vi "WhichGoalVisible.vi"(0 "Goal Measurements":dbl[][](array[numeric]), 1 "No. of Goals":i32) -> (2 "Goal A":cluster{"X":dbl, "Y":dbl, "Dist":dbl}, 3 "Goal B":cluster{"X":dbl, "Y":dbl, "Dist":dbl}, 4 "Goal C":cluster{"X":dbl, "Y":dbl, "Dist":dbl})   [LabVIEW 2015]
uses:
  Robot Global Data.vi
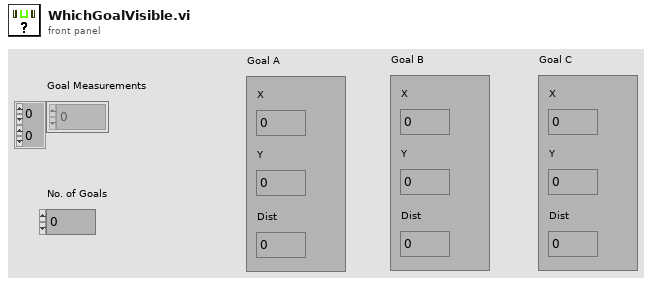
[diagram p1: front panel]
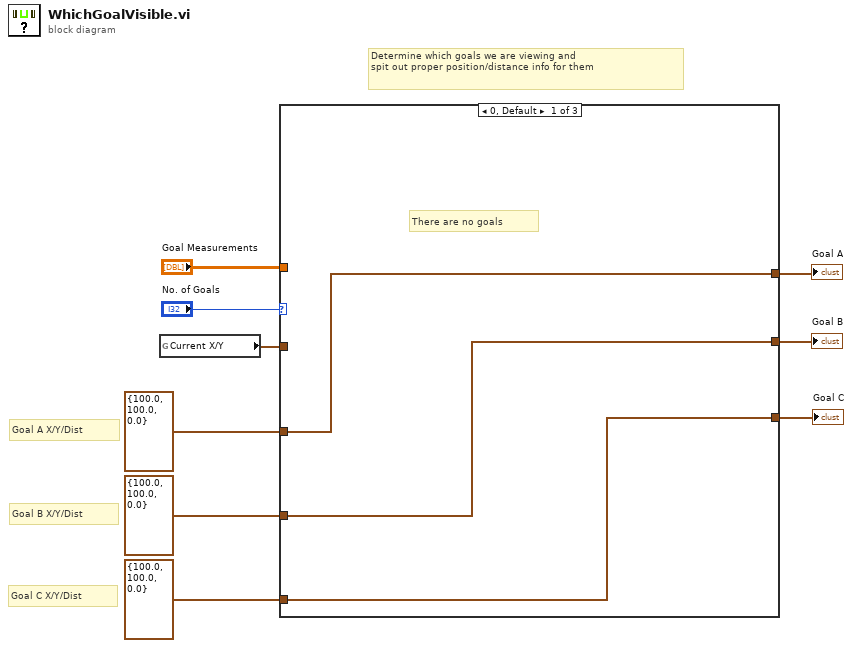
[diagram p0: block diagram]
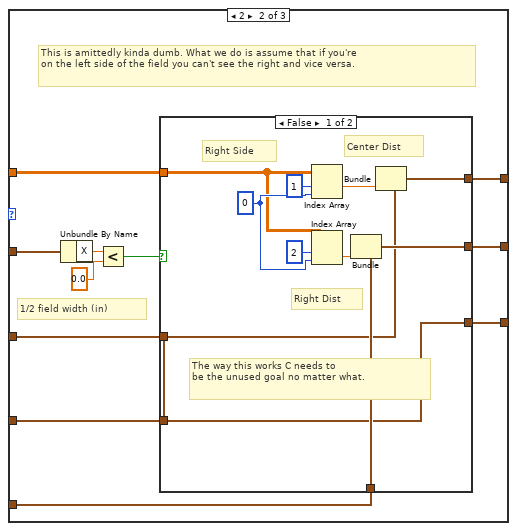
[diagram p2: hidden frame]
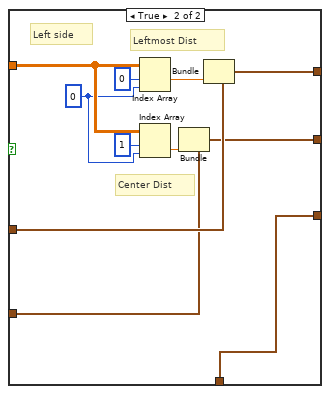
[diagram p3: hidden frame]
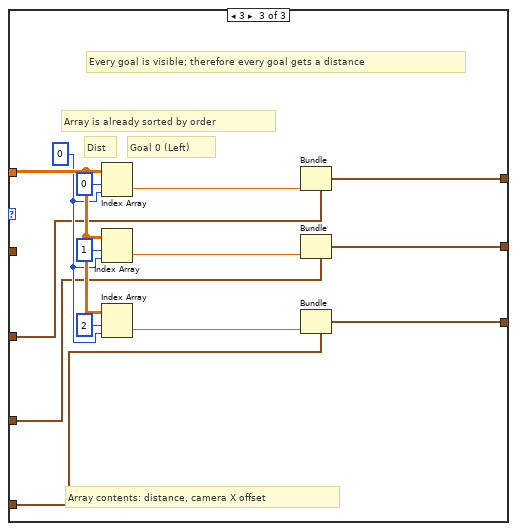
[diagram p4: hidden frame]
diagram:
  # "Determine which goals we are viewing and\nspit out proper position/distance info for them"
  # "Goal C X/Y/Dist"
  # "Goal B X/Y/Dist"
  # "Goal A X/Y/Dist"
  n1 = global read "Robot Global Data.vi" "Current X/Y"() -> (w1:cluster{"X":dbl, "Y":dbl})
  n2 = case shown="0, Default" "No. of Goals" {
    tunnel: [w12 w14 w55] -> w8
    tunnel: [w11 w15 w54] -> w7
    tunnel: [w10 w13 w52] -> w6
    tunnel: "Goal Measurements" -> [_ w16 w58]
    tunnel: cluster{dbl, dbl, dbl} {100.0, 100.0, 0.0} -> [w12 w19 w48]
    tunnel: cluster{dbl, dbl, dbl} {100.0, 100.0, 0.0} -> [w11 w18 w47]
    tunnel: cluster{dbl, dbl, dbl} {100.0, 100.0, 0.0} -> [w10 w17 w46]
    tunnel: w1 -> [_ w23 _]
    frame 0, Default {
      # "There are no goals"
    }
    frame 2 {
      # "This is amittedly kinda dumb. What we do is assume that if you're\non the left side of the field you can't see the right and vice versa."
      # "1/2 field width (in)"
      n3 = Unbundle By Name(w23) -> ("X"=w22:dbl)
      n4 = Less?(x=w22, y=0.0) -> (x < y?=w20:bool)
      n5 = case shown="False" w20 {
        tunnel: w19 -> [_ w40]
        tunnel: w18 -> [w24 w37]
        tunnel: w17 -> [w28 w34]
        tunnel: w16 -> [w27 w44]
        tunnel: [w25 w36] -> w15
        tunnel: [w26 w35] -> w14
        tunnel: [w24 w34] -> w13
        frame False {
          w31 = 0 ("index (row)")
          # "The way this works C needs to\nbe the unused goal no matter what."
          # "Center Dist"
          # "Right Dist"
          # "Right Side"
          n6 = Index Array(array=w27, index (row)=1, index (col)=w31) -> (element=w30:dbl)
          n7 = Index Array(array=w27, index (row)=2, index (col)=w31) -> (element=w29:dbl)
          n8 = Bundle(cluster=w28, w29) -> (w25:cluster{dbl, dbl, dbl})  [unwired: 2 in]
          n9 = Bundle(cluster=w24, w30) -> (w26:cluster{dbl, dbl, dbl})  [unwired: 2 in]
        }
        frame True {
          w41 = 0 ("index (row)")
          # "Center Dist"
          # "Leftmost Dist"
          # "Left side"
          n10 = Index Array(array=w44, index (row)=0, index (col)=w41) -> (element=w39:dbl)
          n11 = Index Array(array=w44, index (row)=1, index (col)=w41) -> (element=w38:dbl)
          n12 = Bundle(cluster=w37, w38) -> (w36:cluster{dbl, dbl, dbl})  [unwired: 2 in]
          n13 = Bundle(cluster=w40, w39) -> (w35:cluster{dbl, dbl, dbl})  [unwired: 2 in]
        }
      }
    }
    frame 3 {
      w49 = 0 ("index (col)")
      # "Every goal is visible; therefore every goal gets a distance"
      # "Goal 0 (Left)"
      # "Dist"
      # "Array contents: distance, camera X offset"
      # "Array is already sorted by order"
      n14 = Index Array(array=w58, index (row)=0, index (col)=w49) -> (element=w45:dbl)
      n15 = Index Array(array=w58, index (row)=1, index (col)=w49) -> (element=w53:dbl)
      n16 = Index Array(array=w58, index (row)=2, index (col)=w49) -> (element=w51:dbl)
      n17 = Bundle(cluster=w48, w45) -> (w55:cluster{dbl, dbl, dbl})  [unwired: 2 in]
      n18 = Bundle(cluster=w47, w53) -> (w54:cluster{dbl, dbl, dbl})  [unwired: 2 in]
      n19 = Bundle(cluster=w46, w51) -> (w52:cluster{dbl, dbl, dbl})  [unwired: 2 in]
    }
  }
  "Goal A" <- w8
  "Goal B" <- w7
  "Goal C" <- w6
